vi "PrinterZT230_NoPLC.vi"(8 "error in":errorcluster, 10 "PN":string="T510587", 11 "PRNfile":path=path "C:/HVAC/Printer/SU2_HVAC_wLOGO.prn") -> (0 "error out":errorcluster, 2 "Result":string)   [LabVIEW 2020]
uses:
  <vilib>/Utility/config.llb/Read Key (String).vi
  <vilib>/Utility/config.llb/NI_LVConfig.lvlib
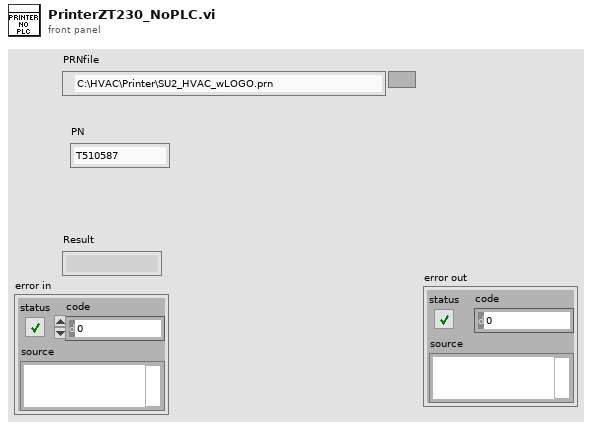
[diagram p1: front panel]
types:
  T1 = enum16{"open", "replace", "create", "open or create", "replace or create", "replace or create with confirmation"}
  T2 = typedef "NI_LVConfig.lvlib/Config Data RefNum.ctl" = refnum<k1>
  T3 = typedef "NewPNConfig.ctl" = cluster{"L/R":u8, "PN":string, "M6_Camera":u16, "Screw 2":u16, "Scanner3_1":string, "Scanner3_2":string, "Scanner7_1":string, "Scanner9_1":string, "Scanner9_2":string, "Scanner11_1":string, "Scanner16_1":string, "Scanner19_1":string, "Scanner3_3":string, "Scanner7_2":string, "Scanner7_3":string, "Scanner9_3":string, "Scanner11_2":string, "Scanner11_3":string, "Scanner16_2":string, "Scanner16_3":string, "Scanner19_2":string, "Scanner19_3":string}
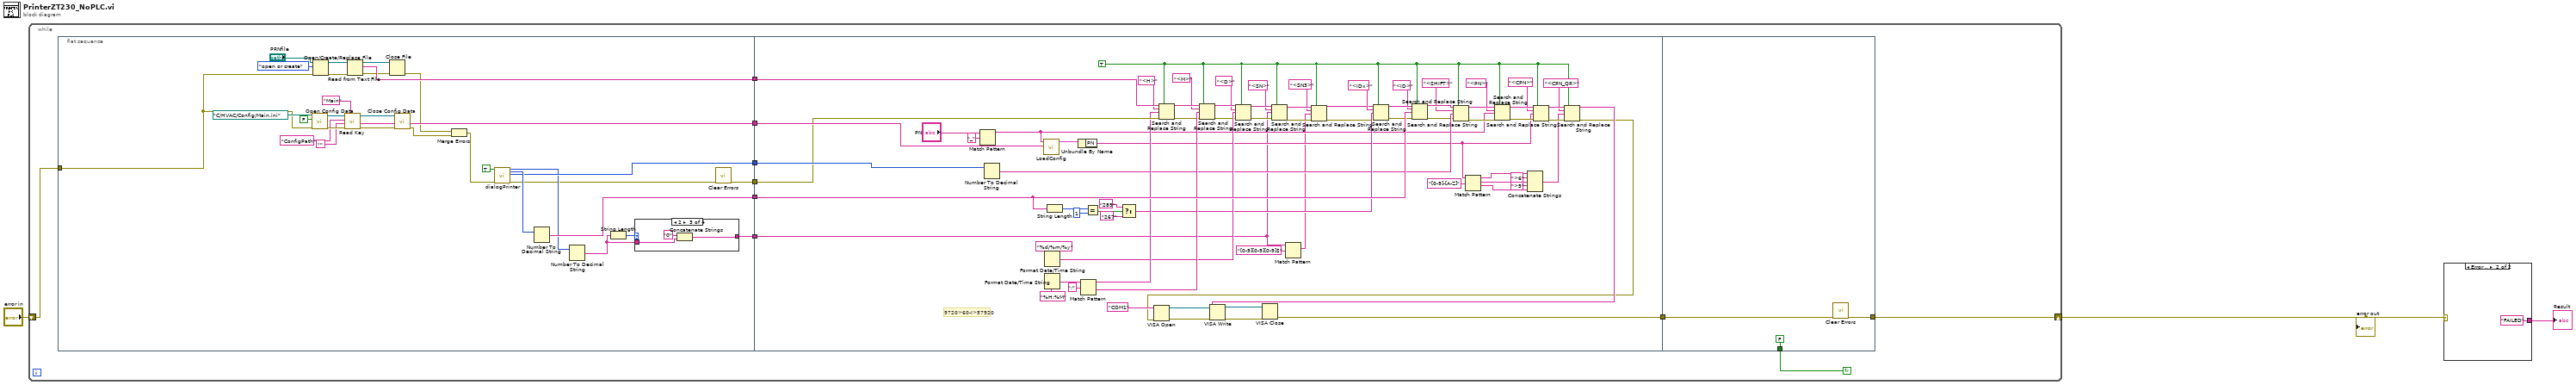
[diagram p0: block diagram]
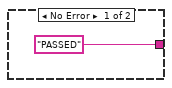
[diagram p2: hidden frame]
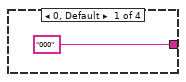
[diagram p3: hidden frame]
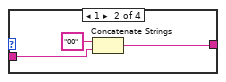
[diagram p4: hidden frame]
diagram:
  n1 = while {
    shift-right: [w7] -> w3
    shift-left: "error in" -> [w4]
    stop <- w8 continue-if-true
    n2 = flat-sequence {
      tunnel: [w44] -> w13
      tunnel: [w43] -> w12
      tunnel: [w21] -> w11
      tunnel: [w42] -> w10
      tunnel: [w41] -> w6
      tunnel: [w17] -> w5
      tunnel: w4 -> [w19]
      tunnel: w13 -> [w126]
      tunnel: w12 -> [w125]
      tunnel: w11 -> [w124]
      tunnel: w10 -> [w123]
      tunnel: [w122] -> w9
      tunnel: w6 -> [w121]
      tunnel: w5 -> [w60]
      tunnel: w9 -> [w128]
      tunnel: [FALSE] -> w8
      tunnel: [w129] -> w7
      frame #0 {
        n3 = call <vilib>:"Open Config Data.vi"("error in (no error)"=w19, "create file if necessary (T)"=FALSE, "configuration file path"=path "C:/HVAC/Config/Main.ini") -> ("error out"=w37:errorcluster, "refnum"=w38:T2)  [unwired: 6 in, 1 out]
        n4 = Open/Create/Replace File(file path (use dialog)="PRNfile", error in=w19, operation (0:open)=T1."open or create") -> (refnum out=w29:refnum<file>, error out=w28:errorcluster)  [unwired: 3 in, 1 out]
        n5 = call-poly <vilib>:"Read Key.vi"("section"="Main", "error in (no error)"=w37, "default value"="", "key"="ConfigPath", "refnum"=w38) -> ("error out"=w39:errorcluster, "value"=w44:string, "refnum out"=w40:T2)  [unwired: 3 in, 1 out]
        n6 = Read from Text File(file (use dialog)=w29, error in=w28) -> (refnum out=w31:refnum<file>, text=w43:string, error out=w30:errorcluster)  [unwired: 2 in, 1 out]
        n7 = Close File(refnum=w31, error in=w30) -> (error out=w24:errorcluster)  [unwired: 1 out]
        n8 = call <vilib>:"Close Config Data.vi"("error in (no error)"=w39, "refnum"=w40) -> ("error out"=w25:errorcluster)  [unwired: 8 in, 1 out]
        n9 = Merge Errors(w24, w25) -> (w15:errorcluster)
        n10 = call "dialogPrinter.vi"("Enable"=TRUE, "error in (no error)"=w15) -> ("SNout"=w20:i16, "ID"=w22:i8, "Shift"=w21:i8, "error out"=w14:errorcluster)  [unwired: 13 in, 1 out]
        n11 = Number To Decimal String(number=w22) -> (decimal integer string=w41:string)  [unwired: 1 in]
        n12 = Number To Decimal String(number=w20) -> (decimal integer string=w18:string)  [unwired: 1 in]
        n13 = String Length(string=w18) -> (length=w23:i32)
        n14 = case shown="2" w23 {
          tunnel: ["000" w48 w51 w52] -> w17
          tunnel: w18 -> [_ w47 w50 w52]
          frame 0, Default {
          }
          frame 1 {
            n15 = Concatenate Strings("00" ("string"), w47) -> (w48:string)
          }
          frame 2 {
            n16 = Concatenate Strings("0" ("string"), w50) -> (w51:string)
          }
          frame 3 {
          }
        }
        n17 = call <vilib>:"Clear Errors.vi"("error in (no error)"=w14) -> ("error out"=w42:errorcluster)  [unwired: 5 in, 1 out]
      }
      frame #1 {
        w55 = TRUE ("replace all? (F)")
        # "9720>60-I>57920"
        n18 = Match Pattern(string="PN", regular expression="_") -> (before substring=w77:string)  [unwired: 1 in, 3 out]
        n19 = Number To Decimal String(number=w124) -> (decimal integer string=w90:string)  [unwired: 1 in]
        n20 = call "LoadConfig.vi"("Path"=w126, "PN"=w77) -> ("Cluster"=w85:T3)  [unwired: 9 in]
        n21 = Format Date/Time String(time format string (%c)="%H:%M") -> (date/time string=w116:string)  [unwired: 2 in]
        n22 = Format Date/Time String(time format string (%c)="%d/%m/%y") -> (date/time string=w106:string)  [unwired: 2 in]
        n23 = String Length(string=w121) -> (length=w101:i32)
        n24 = Unbundle By Name(w85) -> ("PN"=w63:string)
        n25 = Match Pattern(string=w116, regular expression=":") -> (before substring=w111:string, after substring=w108:string)  [unwired: 1 in, 2 out]
        n26 = Equal?(x=w101, y=1) -> (x = y?=w98:bool)
        n27 = Select(t="289", s=w98, f="267") -> (s? t:f=w95:string)
        n28 = Search and Replace String(replace all?=w55, input string=w125, search string="<H>", replace string=w111, error in=w123) -> (result string=w110:string, error out=w84:errorcluster)  [unwired: 3 in, 2 out]
        n29 = Search and Replace String(replace all?=w55, input string=w110, search string="<M>", replace string=w108, error in=w84) -> (result string=w105:string, error out=w83:errorcluster)  [unwired: 3 in, 2 out]
        n30 = Search and Replace String(replace all?=w55, input string=w105, search string="<D>", replace string=w106, error in=w83) -> (result string=w103:string, error out=w82:errorcluster)  [unwired: 3 in, 2 out]
        n31 = Search and Replace String(replace all?=w55, input string=w103, search string="<SN>", replace string=w60, error in=w82) -> (result string=w56:string, error out=w59:errorcluster)  [unwired: 3 in, 2 out]
        n32 = Match Pattern(string=w60, regular expression="[0-9][0-9][0-9]$") -> (match substring=w53:string)  [unwired: 1 in, 3 out]
        n33 = Search and Replace String(replace all?=w55, input string=w56, search string="<SN3>", replace string=w53, error in=w59) -> (result string=w57:string, error out=w58:errorcluster)  [unwired: 3 in, 2 out]
        n34 = Search and Replace String(replace all?=w55, input string=w57, search string="<IDx>", replace string=w95, error in=w58) -> (result string=w94:string, error out=w81:errorcluster)  [unwired: 3 in, 2 out]
        n35 = Search and Replace String(replace all?=w55, input string=w94, search string="<ID>", replace string=w121, error in=w81) -> (result string=w92:string, error out=w80:errorcluster)  [unwired: 3 in, 2 out]
        n36 = Search and Replace String(replace all?=w55, input string=w92, search string="<SHIFT>" ("input string"), replace string=w90, error in=w80) -> (result string=w88:string, error out=w79:errorcluster)  [unwired: 3 in, 2 out]
        n37 = Match Pattern(string=w63, regular expression="[0-9]-[A-Z]") -> (before substring=w66:string, match substring=w67:string, after substring=w68:string)  [unwired: 1 in, 1 out]
        n38 = Search and Replace String(replace all?=w55, input string=w88, search string="<PN>", replace string=w77, error in=w79) -> (result string=w89:string, error out=w78:errorcluster)  [unwired: 3 in, 2 out]
        n39 = Concatenate Strings(w66, ">6" ("string"), w67, ">5" ("string"), w68) -> (w62:string)
        n40 = Search and Replace String(replace all?=w55, input string=w89, search string="<CPN>", replace string=w63, error in=w78) -> (result string=w74:string, error out=w72:errorcluster)  [unwired: 3 in, 2 out]
        n41 = Search and Replace String(replace all?=w55, input string=w74, search string="<CPN_QR>", replace string=w62, error in=w72) -> (result string=w73:string, error out=w71:errorcluster)  [unwired: 3 in, 2 out]
        n42 = VISA Open(error in (no error)=w71, VISA resource name="COM1") -> (VISA resource name=w118:refnum<visa-resource-name>, error out=w119:errorcluster)  [unwired: 3 in]
        n43 = VISA Write(VISA resource name=w118, write buffer=w73, error in (no error)=w119) -> (VISA resource name out=w113:refnum<visa-resource-name>, error out=w114:errorcluster)  [unwired: 1 out]
        n44 = VISA Close(VISA resource name=w113, error in (no error)=w114) -> (error out=w122:errorcluster)
      }
      frame #2 {
        n45 = call <vilib>:"Clear Errors.vi"("error in (no error)"=w128) -> ("error out"=w129:errorcluster)  [unwired: 5 in, 1 out]
      }
    }
  }
  "error out" <- w3
  n46 = case shown="Error .." w3 {
    tunnel: ["PASSED" ("Result") "FAILED" ("Result")] -> w2
    frame No Error {
    }
    frame Error {
    }
  }
  "Result" <- w2
